vi "GetString.vi"() -> (3 "String":string="Hello World!")   [LabVIEW 2015]
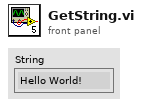
[diagram p1: front panel]
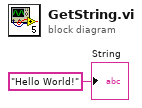
[diagram p0: block diagram]
diagram:
  "String" <- "Hello World!"
